vi "Binning.vi"() -> ()   [LabVIEW 2010]
panel:
  in  "Binning":u32
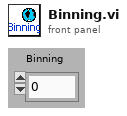
[diagram p1: front panel]
diagram:
